vi "Apply.vi"(8 "error in (no error)":errorcluster, 11 "object in":refnum<class "Fetch Waveforms CFG.lvclass">) -> (0 "error out":errorcluster, 3 "object out":refnum<class "Fetch Waveforms CFG.lvclass">)   [LabVIEW 2023, in "Scope Simulated CFGs.lvlib" / "Fetch Waveforms CFG.lvclass"]
uses:
  Fetch Waveforms CFG.lvclass
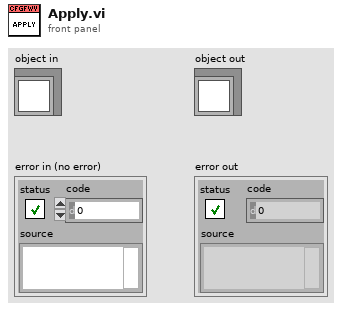
[diagram p1: front panel]
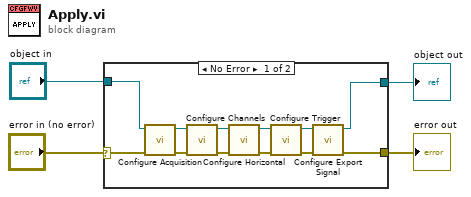
[diagram p0: block diagram]
diagram:
  n1 = case shown="No Error" "error in (no error)" {
    selector: "error in (no error)" -> [w5 w17]
    tunnel: "object in" -> [w8 w18]
    tunnel: [w7 w17] -> w3
    tunnel: [w6 w18] -> w2
    frame No Error {
      n2 = call-dynamic "Configure Acquisition.vi"("error in (no error)"=w5, "object in"=w8) -> ("error out"=w15:errorcluster, "object out"=w16:refnum<class "Fetch Waveforms CFG.lvclass">)  [unwired: 8 in]
      n3 = call-dynamic "Configure Channels.vi"("error in (no error)"=w15, "object in"=w16) -> ("error out"=w14:errorcluster, "object out"=w11:refnum<class "Fetch Waveforms CFG.lvclass">)  [unwired: 8 in]
      n4 = call-dynamic "Configure Horizontal.vi"("error in"=w14, "object in"=w11) -> ("error out"=w13:errorcluster, "object out"=w10:refnum<class "Fetch Waveforms CFG.lvclass">)  [unwired: 8 in]
      n5 = call-dynamic "Configure Trigger.vi"("error in"=w13, "object in"=w10) -> ("error out"=w12:errorcluster, "object out"=w9:refnum<class "Fetch Waveforms CFG.lvclass">)  [unwired: 8 in]
      n6 = call-dynamic "Configure Export Signal.vi"("error in (no error)"=w12, "object in"=w9) -> ("error out"=w7:errorcluster, "object out"=w6:refnum<class "Fetch Waveforms CFG.lvclass">)  [unwired: 8 in]
    }
    frame Error {
    }
  }
  "error out" <- w3
  "object out" <- w2
